vi "DefaultPsTactic.vi"(9 "Game in":refnum<class "Game.lvclass">, 10 "Robot":refnum<class "Robot.lvclass">, 11 "DefaultPsTactic in":refnum<class "DefaultPsTactic.lvclass">) -> (2 "Robot out":refnum<class "Robot.lvclass">, 3 "DefaultPsTactic out":refnum<class "DefaultPsTactic.lvclass">)   [LabVIEW 2020, in "DefaultPsTactic.lvclass"]
uses:
  DefaultPsTactic.lvclass
  C:/Users/User/Documents/GitHub/SSL_AI/Tactic_class/Tactic.lvclass
  Robot_class/Robot.lvclass
  Game_class/Game.lvclass
  Robot_class/tactics.ctl
  Tactic_class/Tactic.lvclass/Tactic.ctl
  Game_class/Game.lvclass/Game.ctl
  Object_class/Object.lvclass/Object.ctl
  Ball_class/Ball.lvclass/Ball.ctl
  Robot_class/Robot.lvclass/Robot.ctl
  Game_class/Read BallRef.vi
  Object_class/Read x.vi
  Ball_class/Read v_x.vi
  Tactic_class/Read Skillbook.vi
  Robot_class/Write tactic.vi
  Ball_class/Ball.lvclass
  C:/Users/User/Documents/GitHub/SSL_AI/Object_class/Object.lvclass
  Skillbook_class/Skillbook.lvclass
  AttackPsSkill_class/AttackPsSkill.lvclass
  DefensePsSkill_class/DefensePsSkill.lvclass
panel:
  out "x .or. y?":bool
  out "error out":errorcluster
  in  "error in (no error)":errorcluster
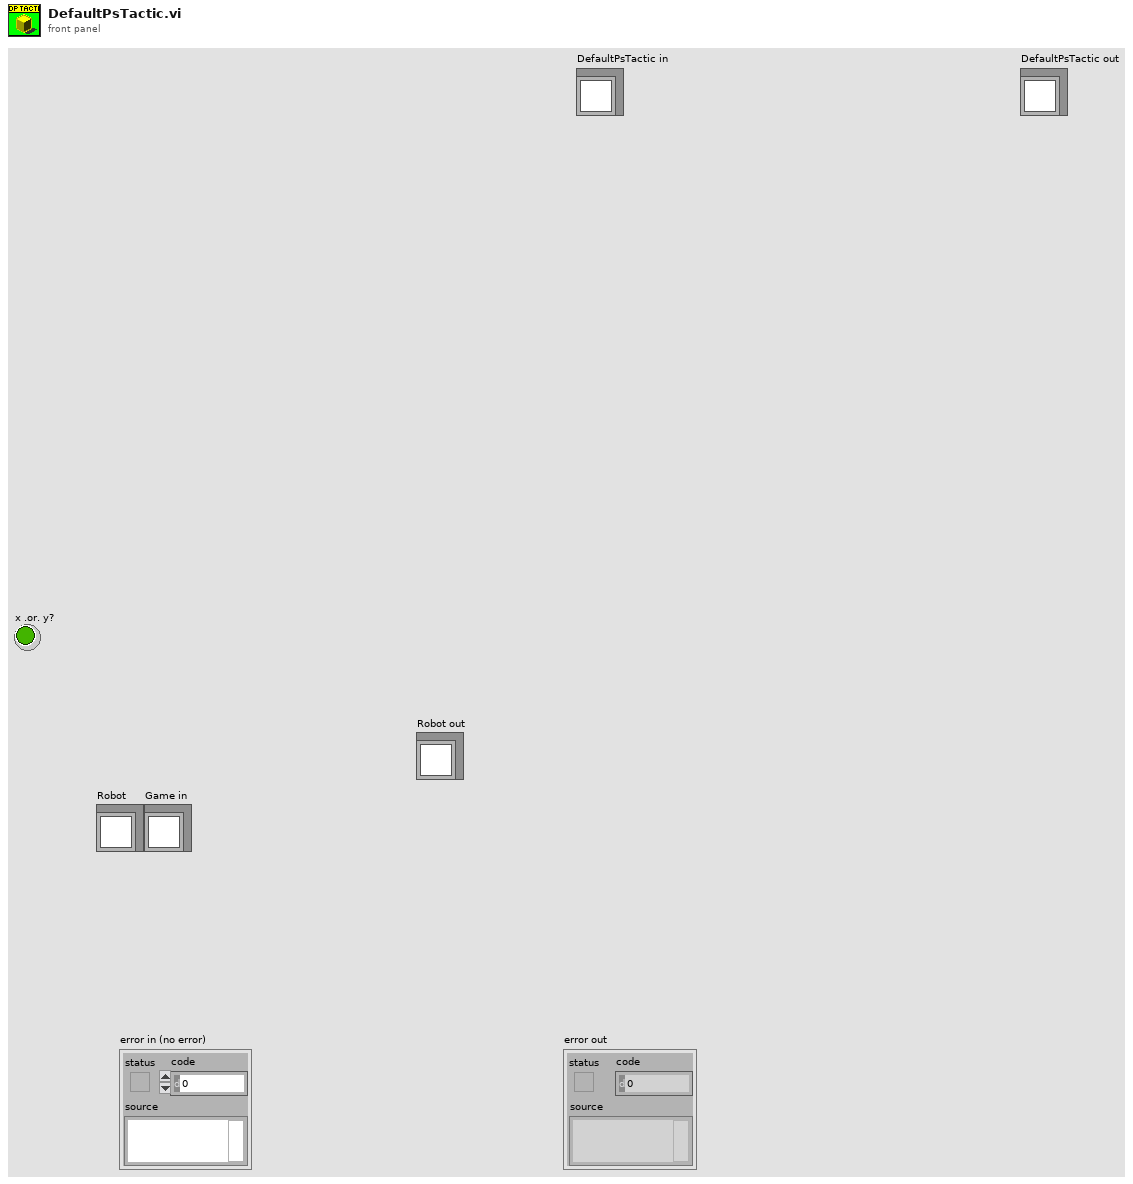
[diagram p1: front panel]
types:
  T1 = typedef "tactics.ctl" = enum16{"PenaltyAttacker", "DefaultPs", "PassObserver", "PenaltyDefense", "Test", "DefendGoal", "Marker", "FollowAttacker", "DefendArea", "Shoot", "AttackerAimGoal", "AttackerBallOutOfField", "AttackerBlock", "AttackerStop", "Duelist", "Halt", "ZigZag", "GoTo", "Timeout", "KickToPassReceiver", "PositionToReceivePass", "PassReceiver", "WaitPass"}
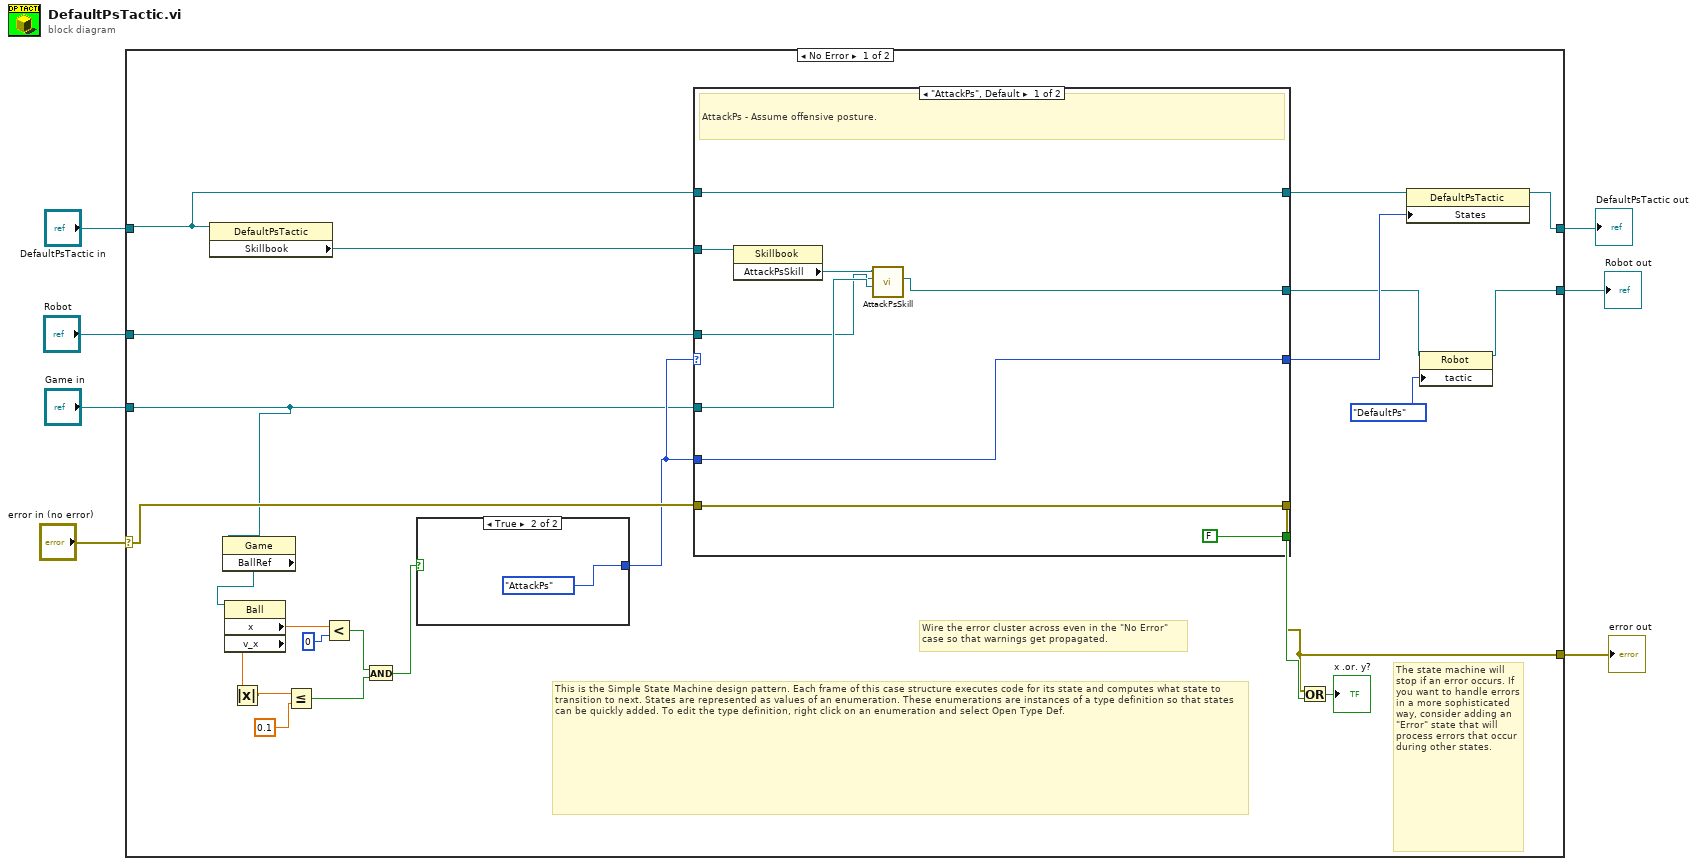
[diagram p0: block diagram]
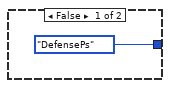
[diagram p2: hidden frame]
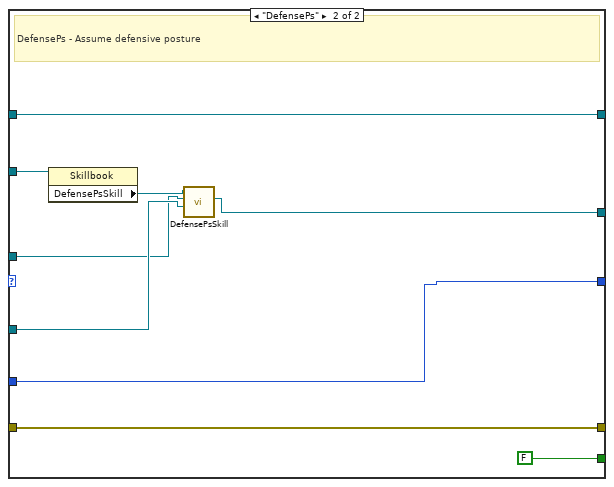
[diagram p3: hidden frame]
diagram:
  n1 = case shown="No Error" "error in (no error)" {
    selector: "error in (no error)" -> [w29 w54]
    tunnel: [w28 w54] -> w6
    tunnel: [w23 w53] -> w2
    tunnel: "DefaultPsTactic in" -> [w26 w53]
    tunnel: "Robot" -> [w27 w52]
    tunnel: [w20 w52] -> w4
    tunnel: "Game in" -> [w17 _]
    frame No Error {
      # "The state machine will stop if an error occurs. If you want to handle errors in a more sophisticated way, consider adding an \"Error\" state that will process errors that occur during other states."
      # "This is the Simple State Machine design pattern. Each frame of this case structure executes code for its state and computes what state to transition to next. States are represented as values of an enumeration. These enumerations are instances of a type definition so that states can be quickly added. To edit the type definition, right click on an enumeration and select Open Type Def."
      # "Wire the error cluster across even in the \"No Error\"\ncase so that warnings get propagated."
      n2 = property class="DefaultPsTactic"(reference=w26) -> ("Skillbook"=w25:refnum<class "Skillbook.lvclass">)  [unwired: 1 in, 2 out]
      n3 = property class="Game"(reference=w17) -> ("BallRef"=w16:refnum<class "Ball.lvclass">)  [unwired: 1 in, 2 out]
      n4 = property class="Ball"(reference=w16) -> ("x"=w11:dbl, "v_x"=w15:dbl)  [unwired: 1 in, 2 out]
      n5 = Absolute Value(x=w15) -> (abs(x)=w14:dbl)
      n6 = Less Or Equal?(x=w14, y=0.1) -> (x <= y?=w9:bool)
      n7 = Less?(x=w11, y=0) -> (x < y?=w10:bool)
      n8 = And(x=w10, y=w9) -> (x .and. y?=w8:bool)
      n9 = case shown="True" w8 {
        tunnel: [enum16{"Exit", "AttackPs", "DefensePs"}."DefensePs" ("States") enum16{"Exit", "AttackPs", "DefensePs"}."AttackPs" ("States")] -> w18
        frame False {
        }
        frame True {
        }
      }
      n10 = case shown="\"AttackPs\", Default" w18 {
        tunnel: [w34 w43] -> w22
        tunnel: [FALSE ("Stop Loop?") FALSE ("Stop Loop?")] -> w31
        tunnel: w29 -> [w41 w50]
        tunnel: [w41 w50] -> w28
        tunnel: w25 -> [w40 w49]
        tunnel: w27 -> [w36 w45]
        tunnel: [w35 w44] -> w21
        tunnel: [w39 w48] -> w24
        tunnel: w26 -> [w39 w48]
        tunnel: w17 -> [w37 w46]
        tunnel: w18 -> [w34 w43]
        frame "AttackPs", Default {
          # "AttackPs - Assume offensive posture."
          n11 = property class="Skillbook"(reference=w40) -> ("AttackPsSkill"=w38:refnum<class "AttackPsSkill.lvclass">)  [unwired: 1 in, 2 out]
          n12 = call "AttackPsSkill.vi"("Game in"=w37, "Robot"=w36, "AttackPsSkill in"=w38) -> ("Robot out"=w35:refnum<class "Robot.lvclass">)  [unwired: 7 in, 1 out]
        }
        frame "DefensePs" {
          # "DefensePs - Assume defensive posture"
          n13 = property class="Skillbook"(reference=w49) -> ("DefensePsSkill"=w47:refnum<class "DefensePsSkill.lvclass">)  [unwired: 1 in, 2 out]
          n14 = call "DefensePsSkill.vi"("Game in"=w46, "Robot"=w45, "DefensePsSkill in"=w47) -> ("Robot out"=w44:refnum<class "Robot.lvclass">)  [unwired: 7 in, 1 out]
        }
      }
      n15 = Or(x=w28, y=w31) -> (x .or. y?=→"x .or. y?":bool)
      n16 = property class="DefaultPsTactic"(reference=w24, "States"=w22) -> (reference out=w23:refnum<class "DefaultPsTactic.lvclass">)  [unwired: 1 in, 1 out]
      n17 = property class="Robot"(reference=w21, "tactic"=tactics."DefaultPs") -> (reference out=w20:refnum<class "Robot.lvclass">)  [unwired: 1 in, 1 out]
    }
    frame Error {
    }
  }
  "DefaultPsTactic out" <- w2
  "error out" <- w6
  "Robot out" <- w4
